vi "photodiode.vi"() -> ()   [LabVIEW 2020]
uses:
  <vilib>/LabVIEW Interface for Arduino/Type Defs/Board Type.ctl
  <vilib>/LabVIEW Interface for Arduino/Type Defs/Pin Mode.ctl
  <vilib>/LabVIEW Interface for Arduino/LabVIEW Interface for Arduino.lvlib
panel:
  out "Waveform Chart":u8(graph)
  in  "Duty Cycle":dbl(knob) scale=0.0..255.0
  in  "stop":bool
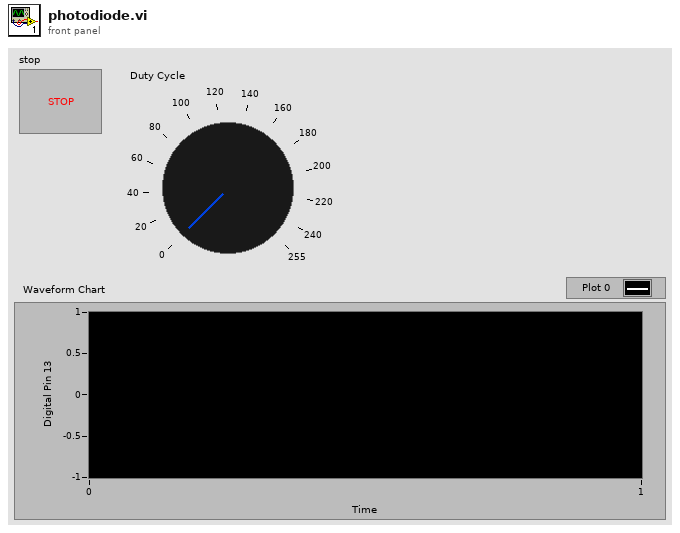
[diagram p1: front panel]
types:
  T1 = typedef "LabVIEW Interface for Arduino.lvlib/Pin Mode.ctl" = enum8{"Input", "Output"}
  T2 = typedef "LabVIEW Interface for Arduino.lvlib/Board Type.ctl" = enum16{"Uno", "Dimuelanove w/Atmega 328", "Mega 2560"}
  T3 = typedef "LabVIEW Interface for Arduino.lvlib/Arduino Resource.ctl" = cluster{"VISA resource":refnum<visa-resource-name>, "Board Type":T2, "Connection Type":enum8{"USB / Serial"}, "Bytes Per Packet (15)":u8}
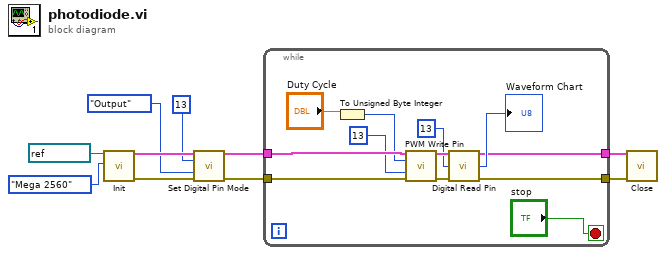
[diagram p0: block diagram]
diagram:
  n1 = call <vilib>:"Init.vi"("VISA resource"=refnum<visa-resource-name> "COM5", "Board Type (Uno)"=Board_Type."Mega 2560") -> ("Arduino Resource"=w8:T3, "error out"=w3:errorcluster)  [unwired: 16 in]
  n2 = call <vilib>:"Set Digital Pin Mode.vi"("Arduino Resource"=w8, "Digital I/O Pin"=u8 13, "Pin Mode (Input)"=Pin_Mode."Output", "error in"=w3) -> ("Arduino Resource"=w5:T3, "error out"=w4:errorcluster)  [unwired: 10 in]
  n3 = while {
    tunnel: w5 -> [w21]
    tunnel: w4 -> [w19]
    tunnel: [w15] -> w2
    tunnel: [w13] -> w1
    stop <- "stop" stop-if-true
    n4 = To Unsigned Byte Integer(number="Duty Cycle") -> (unsigned 8bit integer=w12:u8)
    n5 = call <vilib>:"PWM Write Pin.vi"("Arduino Resource"=w21, "Duty Cycle (0 - 255)"=w12, "PWM Pin (3)"=u8 13, "error in"=w19) -> ("Arduino Resource"=w18:T3, "error out"=w16:errorcluster)  [unwired: 10 in]
    n6 = call <vilib>:"Digital Read Pin.vi"("Arduino Resource"=w18, "Digital I/O Pin (0)"=u8 13, "error in"=w16) -> ("Arduino Resource"=w13:T3, "Value"=→"Waveform Chart":u8, "error out"=w15:errorcluster)  [unwired: 10 in]
  }
  n7 = call <vilib>:"Close.vi"("Arduino Resource"=w1, "error in"=w2) -> ()  [unwired: 13 in, 1 out]
